vi "Dashboard Main.vi"() -> ()   [LabVIEW 2015]
uses:
  <vilib>/Utility/miscctls.llb/LVRowAndColumnTypeDef.ctl
  <vilib>/event_ctls.llb/eventvkey.ctl
  <vilib>/Rock Robotics/WPI/Dashboard/WPI_DashboardLogging Global.vi
  <vilib>/Rock Robotics/Network Tables/NT Read Boolean.vi
  <vilib>/Rock Robotics/Network Tables/NT Read Numeric Array.vi
  <vilib>/Utility/config.llb/Write Key (String).vi
  <vilib>/Utility/config.llb/Write Key (I32).vi
  <vilib>/Utility/config.llb/NI_LVConfig.lvlib
panel:
  in  "TCP":refnum<k5>
  in  "Rec Mode":enum32{"Stop", "Record", "Playback"}(radio)
  in  "Vision":u16(ring) items=["Camera Off", "USB Camera SW", "USB Camera HW", "IP Camera"]
  out "Camera IP":string
  out "Image Message":string="Timeout in Camera Communications"
  in  "Dashboard Tab":T1(tab)
  in  "Select Auto":string(combo)
  out "NT Connection":bool
  in  "Camera Settings":T2={"Frame Rate"=30, "Compression"=30, "Size"=1} {"Frame Rate" scale=1.0..30.0; "Size" items=["640x480", "320x240", "160x120"]}
  out "MotorChart R":cluster{"Numeric":dbl, "Numeric":dbl}(graph)
  out "MotorChart L":T3(graph)
  out "MotorSliders R":cluster{"MotorSlide1":dbl, "MotorSlide2":dbl} {"MotorSlide2" scale=-1.0..1.0 scale format="%#_2e"; "MotorSlide1" scale=-1.0..1.0 scale format="%#_2e"}
  out "MotorSliders L":T4 {"MotorSlide4 2" scale=0.0..14.0 scale format="%#_2e"; "MotorSlide2" scale=-1.0..1.0 scale format="%#_2e"; "MotorSlide1" scale=-1.0..1.0 scale format="%#_2e"}
  out "JS1 Z":dbl(slide) scale=-1.0..1.0 scale format="%#_2e"
  out "JS1 Graph":cluster{"X":dbl, "Y":dbl}[](graph)
  out "JS1 Buttons":T5
  out "JS2 Z":dbl(slide) scale=-1.0..1.0 scale format="%#_2e"
  out "JS2 Graph":cluster{"X":dbl, "Y":dbl}[](graph)
  out "JS2 Buttons":T5
  out "Mode":T6(ring)=enum."Auto Disabled"
  in  "DB Camera Config":bool
  out "fps":dbl format="%#.1g"
  out "Mbps":dbl format="%#.1g"
  out "Mbps LED":bool
  out "Accelerometre/temps":dbl(graph)
  in  "DB/String 9":string
  in  "DB/String 8":string
  in  "DB/String 7":string
  in  "DB/String 6":string
  in  "DB/String 5":string
  in  "DB/String 4":string
  in  "DB/String 3":string
  in  "DB/String 2":string
  in  "DB/String 1":string
  in  "DB/String 0":string
  in  "DB/Slider 0":dbl(slide) scale=0.0..5.0
  in  "DB/Slider 1":dbl(slide) scale=0.0..5.0
  in  "DB/Slider 2":dbl(slide) scale=0.0..5.0
  in  "DB/Slider 3":dbl(slide) scale=0.0..5.0
  out "DB/LED 3":bool
  out "DB/LED 2":bool
  out "DB/LED 1":bool
  out "DB/LED 0":bool
  in  "DB/Button 3":bool
  in  "DB/Button 2":bool
  in  "DB/Button 1":bool
  in  "DB/Button 0":bool caption="New Name"
  out "Voltage Right2":dbl
  out "Voltage Right1":dbl
  out "Voltage Left2":dbl
  out "Voltage Left1":dbl
  in  "vitesse gauche":dbl
  in  "temps de changement de direction":dbl=2.0
  in  "temps pleine vitesse":dbl=1.0
  in  "vitesse droit":dbl
  out "gauche rapide 2":bool
  out "gauche fort 2":bool
  out "droit rapide 2":bool
  out "droit fort  2":bool
  in  "Test Slider":dbl(slide) scale=0.0..100.0 scale format="%#_3g"
  in  "On/Off":bool caption="Solenoid"
  in  "Test Name":u16(ring) items=["Select the test to run..."]
  in  "Test Tree":string(tree)
  in  "Motor":cluster{"Value":dbl, "Enable":bool} {"Value" scale=-1.0..1.0 scale format="%#_3g"}
  out "Progress":T7 {"Test Progress" scale=0.0..100.0}
  in  "Rev/Fwd":cluster{"Forward":bool, "Reverse":bool}
  in  "Test Ring":u16(ring) items=["Monochrome", "Color"]
  out "Cmd Status":string
  in  "Execute Command":bool
  in  "Command Params":string[][](table)
  in  "Command Selection":i32(listbox)
  in  "CheckList":i32(listbox)
  out "Tree":string(tree)
  out "Camera Image":T8(plugin-control)
  out "Background":bool
  # "Left"
  # "Front"
  # "Right"
  # "Battery"
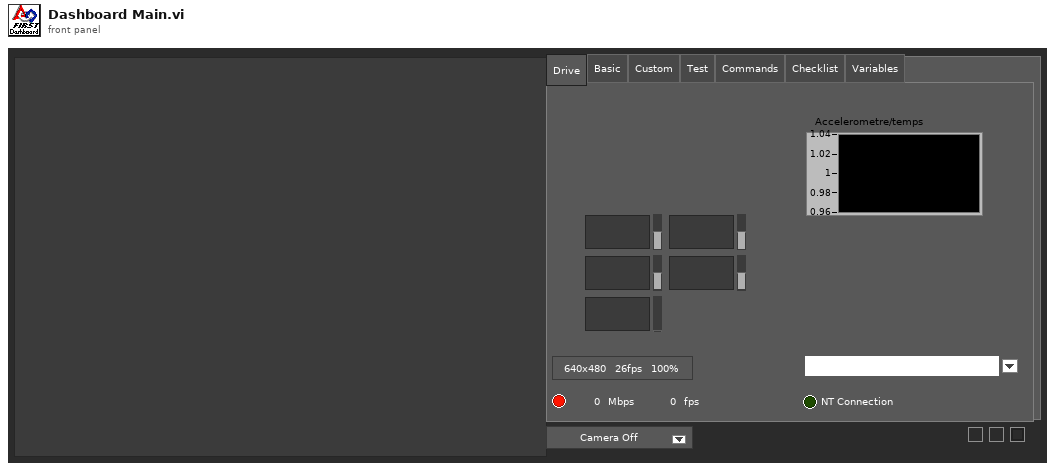
[diagram p1: front panel]
types:
  T1 = enum32{"Drive", "Basic", "Custom", "Test", "Commands", "Checklist", "Variables"}
  T2 = cluster{"Frame Rate":i32, "Compression":i32, "Size":u16}
  T3 = cluster{"Numeric":dbl, "Numeric":dbl, "Battery V":dbl}
  T4 = cluster{"MotorSlide1":dbl, "MotorSlide2":dbl, "MotorSlide4 2":dbl}
  T5 = cluster{bool, bool, bool, bool, bool, bool, bool, bool, bool, bool, bool, bool}
  T6 = enum8{"Tele-Op Disabled", "Tele-Op Enabled", "Auto Disabled", "Auto Enabled", "Test Disabled", "Test Enabled", "Disconnected", "No Code", "E-Stop"}
  T7 = cluster{"Test Progress":u8, "Test Progress Text":string}
  T8 = typedef "IMAQ Image.ctl" = refnum<image>
  T9 = cluster{"IDs":cluster{"RPC field ID":u16, "Unique ID":u16}, "String":string}
  T10 = enum32{"Drive", "Basic", "Custom", "Test", "Checklist", "Variables"}
  T11 = typedef "Image Type" = u32
  T12 = cluster{"Camera Image":refnum<vi>, "Dashboard Tab":refnum<vi>, "Background":refnum<vi>, "Vision":refnum<vi>, "Rec Mode":refnum<vi>, "Test Slider":refnum<vi>, "On/Off ":refnum<vi>, "Test Ring":refnum<vi>, "Rev/Fwd":refnum<vi>, "Test Name":refnum<vi>, "Motor":refnum<vi>, "Progress":refnum<vi>, "CheckList":refnum<vi>, "Tree":refnum<vi>, "Test Tree":refnum<vi>, "Command Params":refnum<vi>, "Command Selection":refnum<vi>, "Execute Command":refnum<vi>, "Cmd Status":refnum<vi>}
  T13 = cluster{"Error Strings":string, "Disable Counts":cluster{u16, u16}, "Rail Faults":cluster{u16, u16, u16}, "Robot IP":string, "DB Mode":u8, "Event Info":cluster{"Name":string, "Type":u8, "Number":u16, "Replay":u8}, "Camera Addr":string}
  T14 = cluster{"Storage":cluster{"Disk Free":u64, "RAM Block":u32, "RAM free":u32}, "CPU Utilization":cluster{"CPU % ISR":sgl, "CPU % Time Crit":sgl, "CPU % Timed Str":sgl, "CPU % High":sgl, "CPU % Above":sgl, "CPU % Normal":sgl, "CPU % Low":sgl}, "CAN":cluster{"% Bus Utilization":sgl, "Bus Off Cnt":u32, "TX_FIFO Full Cnt":u32, "Receive Error Cnt":u8, "Transmit Error Cnt":u8}, "HID":cluster{"HID Outputs":u32, "Rumble Low":u16, "Rumble High":u16}[]}
  T15 = cluster{"Status bits":cluster{"Test Mode":bool, "Autonomous":bool, "Enabled":bool, "Code Start":bool, "Brownout":bool, "Reserved 2":bool, "Reserved 3":bool, "E-Stop":bool}, "Code Trace":cluster{"Disabled":bool, "TeleOp":bool, "Auto":bool, "Test":bool}, "Controller Type":enum16{"unknown", "cRIO", "roboRio"}, "Code?":enum16{"unknown", "noCode", "code"}, "Battery V":dbl}
  T16 = cluster{"Control Bits":cluster{"TestMode":bool, "Autonomous":bool, "Enabled":bool, "FMS Present":bool, bool, bool, bool, "E-Stop":bool}, "Team Station ":u8, "Countdown":sgl, "Joystick Values":cluster{"Axes":dbl[], "Buttons":bool[], "POVs":i16[]}[]}
  T17 = cluster{"Axes":dbl[], "Buttons":bool[], "POVs":i16[]}[]
  T18 = cluster{"Axes":dbl[], "Buttons":bool[], "POVs":i16[]}
  T19 = cluster{"Buttons[0]":bool, "Buttons[1]":bool, "Buttons[2]":bool, "Buttons[3]":bool, "Buttons[4]":bool, "Buttons[5]":bool, "Buttons[6]":bool, "Buttons[7]":bool, "Buttons[8]":bool, "Buttons[9]":bool, "Buttons[10]":bool, "Buttons[11]":bool}
  T20 = typedef "NI_LVConfig.lvlib/Config Data RefNum.ctl" = refnum<k1>
  T21 = cluster{"Operation":enum16{"Update", "Clear"}, "Color Box":u32}[]
  T22 = typedef "eventvkey.ctl" = enum16{"ASCII", "Enter", "Return", "Shift", "Ctrl", "Alt", "Cmd", "Opt", "Caps", "NumLock", "Clear", "Break", "Up", "Down", "Left", "Right", "Insert", "Delete", "Home", "End", "PageUp", "PageDown", "Escape", "Help", "Pause", "ScrollLock", "F1", "F2", "F3", "F4", "F5", "F6", "F7", "F8", "F9", "F10", "F11", "F12", "F13", "F14", "F15", "F16", "F17", "F18", "F19", "F20", "F21", "F22", "F23", "F24", "Play", "VolumeUp", "VolumeDown", "Mute", "Two Byte Char"}
  T23 = cluster{"Image Size":bool, "Image Type":bool, "Pixel Value":bool, "ROI Information":bool, "Zoom Factor":bool}
  T24 = enum8{"Enabled", "Disabled", "Disabled and Grayed Out"}
  T25 = cluster{"Operation":enum16{"Update", "Clear"}, "Color Box":u32}
  T26 = typedef "LVRowAndColumnTypeDef.ctl" = cluster{"Row":i32, "Column":i32}
  T27 = cluster{"Shift":bool, "Ctrl":bool, "Alt":bool, "Cmd":bool, "Opt":bool}
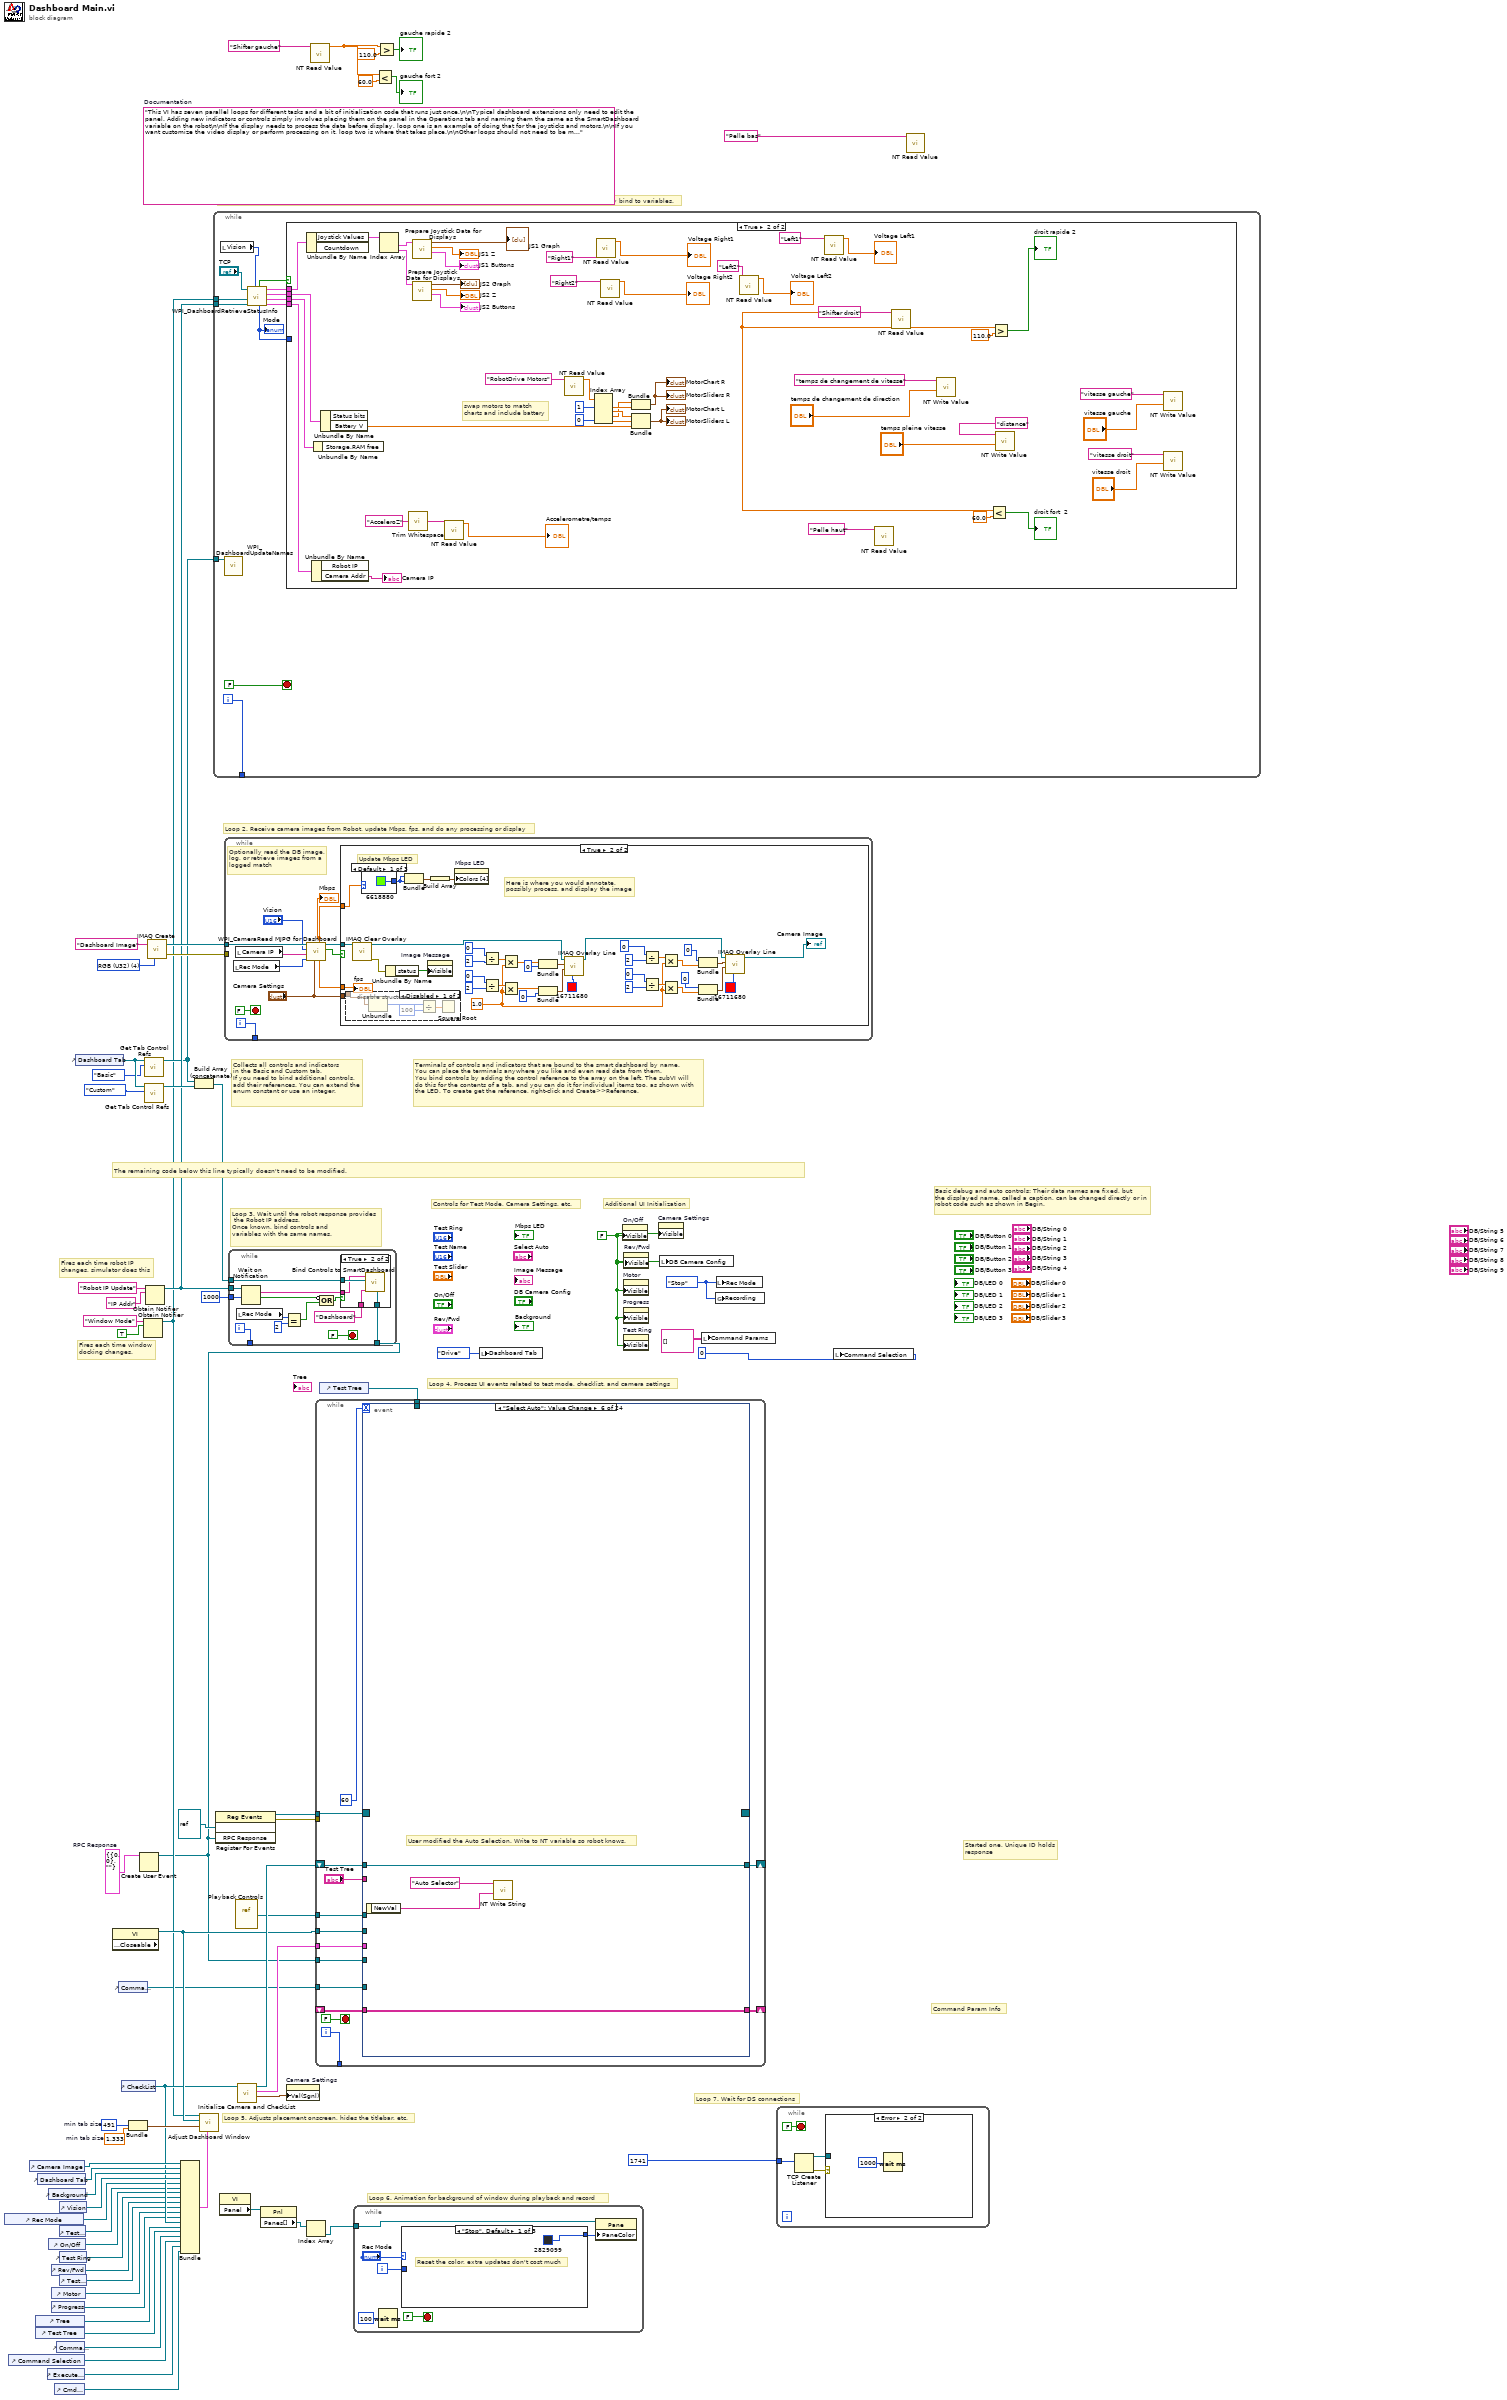
[diagram p0: block diagram]
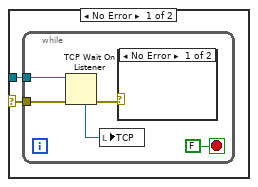
[diagram p2: hidden frame]
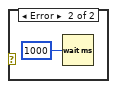
[diagram p3: hidden frame]
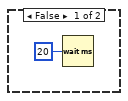
[diagram p4: hidden frame]
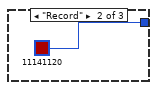
[diagram p5: hidden frame]
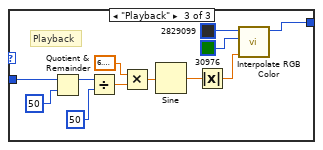
[diagram p6: hidden frame]
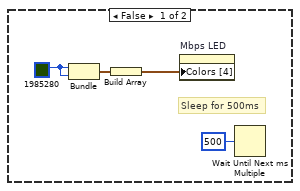
[diagram p8: hidden frame]
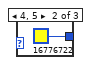
[diagram p10: hidden frame]
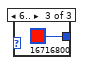
[diagram p11: hidden frame]
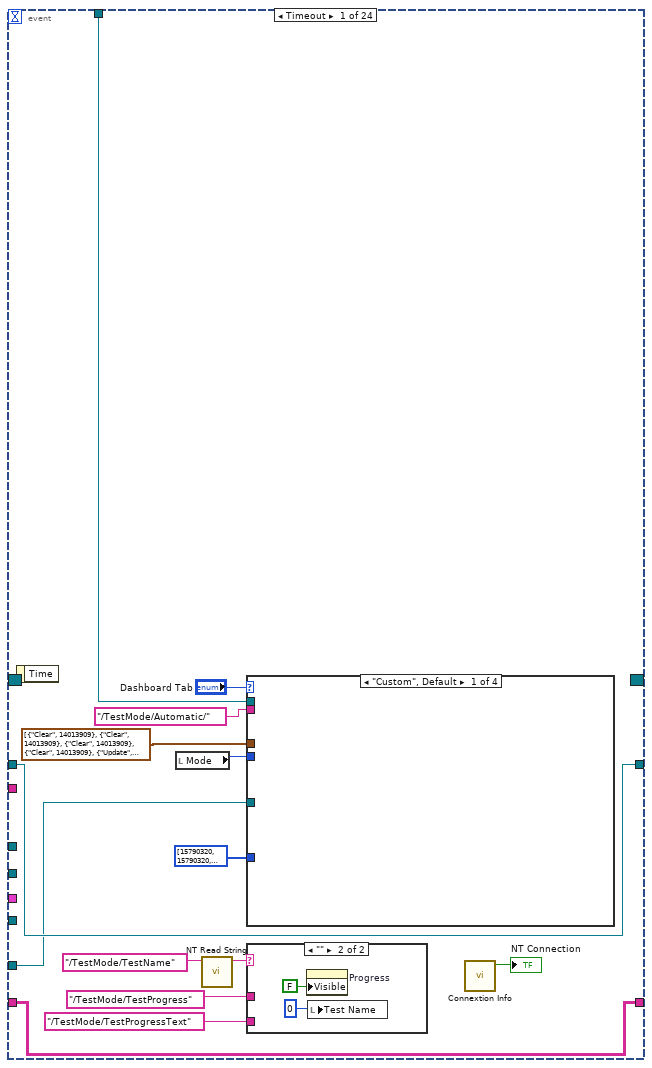
[diagram p12: hidden frame]
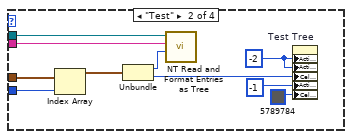
[diagram p13: hidden frame]
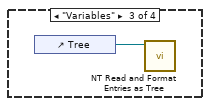
[diagram p14: hidden frame]
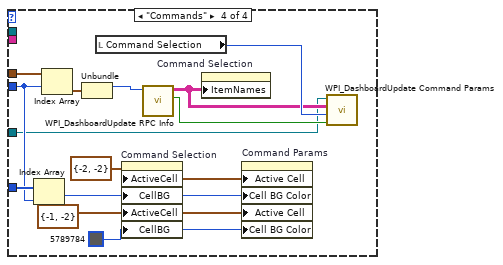
[diagram p15: hidden frame]
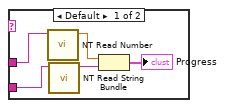
[diagram p16: hidden frame]
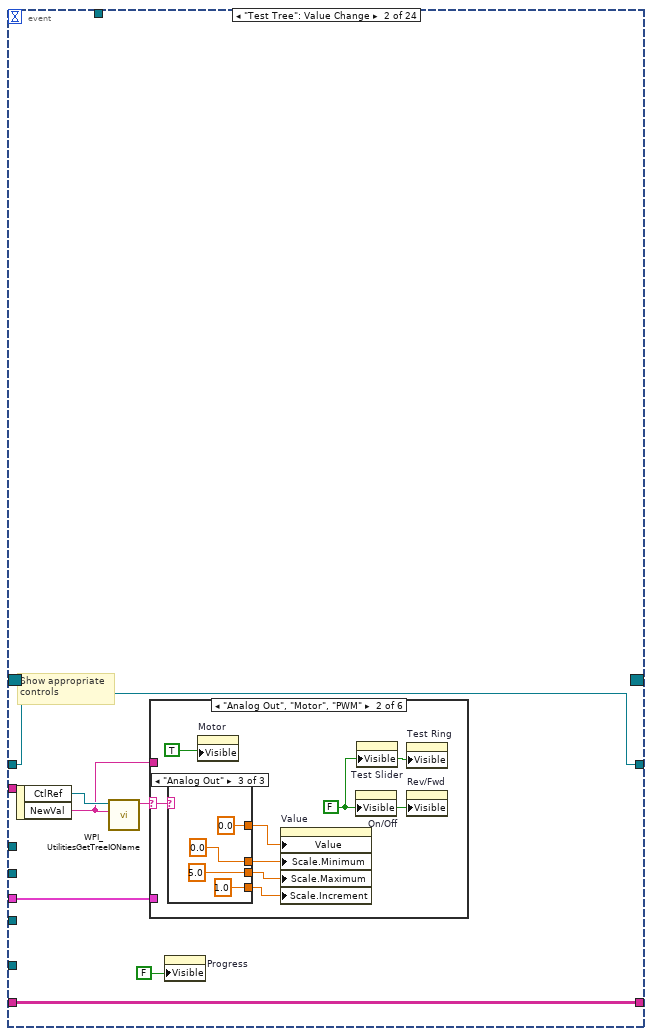
[diagram p17: hidden frame]
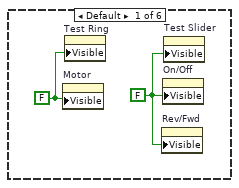
[diagram p18: hidden frame]
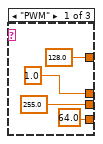
[diagram p19: hidden frame]
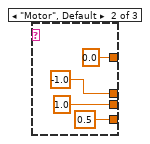
[diagram p20: hidden frame]
diagram:
  w14 = T9 {"IDs"={"RPC field ID"=0, "Unique ID"=0}, "String"=""}  # RPC Response
  w40 = 491  # min tab size
  w39 = 1.333  # min tab size
  w48 = enum32{"Stop", "Record", "Playback"}."Stop" ("Rec Mode")
  w22 = FALSE ("Visible")
  (unwired) "This VI has seven parallel loops for different tasks and a bit of initialization code that runs just once.\n\nTypical dashboard extensions only need to edit the panel. Adding new indicators or controls simply involves placing them on the panel in the Operations tab and naming them the same as the SmartDashboard variable on the robot\n\nIf the display needs to process the data before display, loop one is an example of doing that for the joysticks and motors.\n\nIf you want customize the video display or perform processing on it, loop two is where that takes place.\n\nOther loops should not need to be modified. They are pretty standard, and document the task they perform."  # Documentation
  w68 = T11 4 items=["Grayscale (U8)", "Grayscale (I16)", "Grayscale (SGL)", "Complex (CSG)", "RGB (U32)", "HSL (U32)", "RGB (U64)"] ("Image Type")
  # "Command Param Info"
  # "Started one, Unique ID holds\nresponse"
  # "Loop 7. Wait for DS connections"
  # "Basic debug and auto controls: Their data names are fixed, but\nthe displayed name, called a caption, can be changed directly or in\nrobot code such as shown in Begin."
  # "Controls for Test Mode, Camera Settings, etc."
  # "Additional UI Initialization"
  # "Loop 6. Animation for background of window during playback and record"
  # "Fires each time robot IP\nchanges, simulator does this"
  # "Fires each time window\ndocking changes."
  # "Collects all controls and indicators\nin the Basic and Custom tab.\nIf you need to bind additional controls,\nadd their references. You can extend the\nenum constant or use an integer."
  # "The remaining code below this line typically doesn't need to be modified."
  # "Loop 4. Process UI events related to test mode, checklist, and camera settings"
  # "Terminals of controls and indicators that are bound to the smart dashboard by name.\nYou can place the terminals anywhere you like and even read data from them.\nYou bind controls by adding the control reference to the array on the left. The subVI will\ndo this for the contents of a tab, and you can do it for individual items too, as shown with\nthe LED. To create get the reference, right-click and Create>>Reference."
  # "Loop 3. Wait until the robot response provides\n the Robot IP address.\nOnce known, bind controls and\nvariables with the same names."
  # "Loop 5. Adjusts placement onscreen, hides the titlebar, etc."
  # "Loop 1. Receive various data streams from Driver Station, update joystick, motors, and more complex displays that don't easily bind to variables."
  # "Loop 2. Receive camera images from Robot, update Mbps, fps, and do any processing or display"
  n1 = control-ref of="Rec Mode"() -> (w28:refnum<vi>)
  n2 = control-ref of="Command Selection"() -> (w13:refnum<vi>)
  n3 = control-ref of="Camera Image"() -> (w43:refnum<vi>)
  n4 = control-ref of="Tree"() -> (w32:refnum<vi>)
  n5 = control-ref of="Test Tree"() -> (w31:refnum<vi>)
  n6 = control-ref of="Dashboard Tab"() -> (w42:refnum<vi>)
  n7 = control-ref of="Execute Command"() -> (w15:refnum<vi>)
  n8 = control-ref of="Background"() -> (w37:refnum<vi>)
  n9 = control-ref of="On/Off"() -> (w26:refnum<vi>)
  n10 = control-ref of="Progress"() -> (w23:refnum<vi>)
  n11 = control-ref of="Rev/Fwd"() -> (w24:refnum<vi>)
  n12 = control-ref of="Motor"() -> (w29:refnum<vi>)
  n13 = control-ref of="Cmd Status"() -> (w9:refnum<vi>)
  n14 = control-ref of="Command Params"() -> (w16:refnum<vi>)
  n15 = control-ref of="Test Slider"() -> (w27:refnum<vi>)
  n16 = control-ref of="Vision"() -> (w41:refnum<vi>)
  n17 = control-ref of="Test Ring"() -> (w25:refnum<vi>)
  n18 = control-ref of="Test Name"() -> (w30:refnum<vi>)
  n19 = control-ref of="Dashboard Tab"() -> (w46:refnum<vi>)
  n20 = property class="VI" props=["Front Panel.Closeable"]() -> (reference out=w47:refnum<vi>)  [unwired: 2 in, 2 out]
  n21 = control-ref of="Command Params"() -> (w8:refnum<vi>)
  n22 = control-ref of="CheckList"() -> (w33:refnum<vi>)
  n23 = Bundle("min tab size"=w40, "min tab size"=w39) -> (w38:cluster{"min tab size":i32, "min tab size":dbl})  [unwired: 1 in]
  n24 = Create User Event(user event datatype=w14) -> (user event=w10:refnum<user-event>)  [unwired: 1 in, 1 out]
  n25 = Obtain Notifier(name (unnamed)="Window Mode", notification data type=TRUE) -> (notifier out=w19:refnum<notifier>)  [unwired: 2 in, 2 out]
  n26 = call <vilib>:"Get Tab Control Refs.vi"("Page Index"=T10."Basic" ("Dashboard Tab"), "TabControl in"=w46) -> ("ControlsOnPage"=w20:refnum<vi>[])  [unwired: 9 in]
  n27 = call <vilib>:"Get Tab Control Refs.vi"("Page Index"=T10."Custom" ("Dashboard Tab"), "TabControl in"=w46) -> ("ControlsOnPage"=w45:refnum<vi>[])  [unwired: 9 in]
  n28 = Obtain Notifier(name (unnamed)="Robot IP Update", notification data type="IP Addr" ("name (unnamed)")) -> (notifier out=w21:refnum<notifier>)  [unwired: 2 in, 2 out]
  n29 = call "IMAQ Create"("Image Name"="Dashboard Image", "Image Type"=w68) -> ("New Image"=w66:T8, "error out"=w65:errorcluster)  [unwired: 2 in, 1 out]
  n30 = Bundle("Camera Image"=w43, "Dashboard Tab"=w42, "Background"=w37, "Vision"=w41, "Rec Mode"=w28, "Test Slider"=w27, "On/Off"=w26, "Test Ring"=w25, "Rev/Fwd"=w24, "Test Name"=w30, "Motor"=w29, "Progress"=w23, "CheckList"=w33, "Tree"=w32, "Test Tree"=w31, "Command Params"=w16, "Command Selection"=w13, "Execute Command"=w15, "Cmd Status"=w9) -> (w34:T12)  [unwired: 1 in]
  n31 = Build Array (concatenate)(w20, w45) -> (w44:refnum<vi>[])
  n32 = call "Adjust Dashboard Window.vi"("Sizing Refnums"=w34, "Size Constraints"=w38, "VI"=w47, "WIn Mode"=w19) -> ()  [unwired: 8 in]
  n33 = while {
    tunnel: [w80] -> _
    tunnel: w21 -> [w74]
    tunnel: w20 -> [w73]
    tunnel: w19 -> [w69]
    i -> [w80]
    stop <- FALSE stop-if-true
    n34 = local read "Vision"() -> (w71:u16)
    n35 = call <vilib>:"WPI_DashboardUpdateNames.vi"("Controls on Tab"=w73) -> ()  [unwired: 11 in]
    n36 = call <vilib>:"WPI_DashboardRetrieveStatusInfo.vi"("Vision"=w71, "Binding Refnum"=w74, "Window Mode Notifier"=w69, "TCP Cnx"="TCP") -> ("Power and Errors"=w75:T13, "Robot Metrics"=w78:T14, "Status Info"=w79:T15, "Control Info"=w76:T16, "Robot Mode"=w72:T6, "Process?"=w77:bool)  [unwired: 2 in]
    "Mode" <- w72
    n37 = case shown="True" w77 {
      tunnel: w79 -> [_ w133]
      tunnel: w78 -> [_ w132]
      tunnel: w76 -> [_ w131]
      tunnel: w75 -> [_ w130]
      tunnel: w72 -> [_ _]
      frame False {
        n38 = Wait (ms)(milliseconds to wait=u32 20) -> ()  [unwired: 1 out]
      }
      frame True {
        # "swap motors to match\ncharts and include battery"
        n39 = Unbundle By Name(w131) -> ("Joystick Values"=w120:T17)  [unwired: 1 out]
        n40 = Unbundle By Name(w130) -> ("Camera Addr"=→"Camera IP":string)  [unwired: 1 out]
        n41 = Unbundle By Name(w132) -> ()  [unwired: 1 out]
        n42 = Unbundle By Name(w133) -> ("Battery V"=w121:dbl)  [unwired: 1 out]
        n43 = Index Array(array=w120) -> (element #1=w119:T18, element #2=w114:T18)  [unwired: 2 in]
        n44 = call <vilib>:"Trim Whitespace.vi"("string"="AcceleroZ") -> ("trimmed string"=w93:string)  [unwired: 1 in]
        n45 = call "Prepare Joystick Data for Displays.vi"("Joystick Values"=w114) -> ("Buttons"=→"JS2 Buttons":T19, "Z Axis"=→"JS2 Z":dbl, "Cartesian Data"=→"JS2 Graph":cluster{"X axis":dbl, "X axis":dbl}[])  [unwired: 8 in]
        n46 = call "Prepare Joystick Data for Displays.vi"("Joystick Values"=w119) -> ("Buttons"=→"JS1 Buttons":T19, "Z Axis"=→"JS1 Z":dbl, "Cartesian Data"=→"JS1 Graph":cluster{"X axis":dbl, "X axis":dbl}[])  [unwired: 8 in]
        n47 = call-poly <vilib>:"NT Read Value.vi"("Name"=w93) -> ("Numeric"=→"Accelerometre/temps":dbl)  [unwired: 9 in, 1 out]
        n48 = call-poly <vilib>:"NT Read Value.vi"("Name"="RobotDrive Motors") -> ("Numeric Array"=w109:dbl[])  [unwired: 9 in, 1 out]
        n49 = Index Array(array=w109, index #1=1, index #4=0) -> (element #1=w125:dbl, element #2=w126:dbl, element #3=w124:dbl, element #4=w129:dbl)  [unwired: 2 in]
        n50 = call-poly <vilib>:"NT Read Value.vi"("Name"="Right1") -> ("Numeric"=→"Voltage Right1":dbl)  [unwired: 9 in, 1 out]
        n51 = call-poly <vilib>:"NT Read Value.vi"("Name"="Right2") -> ("Numeric"=→"Voltage Right2":dbl)  [unwired: 9 in, 1 out]
        n52 = Bundle("Numeric"=w124, "Numeric"=w125) -> (→"MotorChart R" →"MotorSliders R":cluster{"Numeric":dbl, "Numeric":dbl})  [unwired: 1 in]
        n53 = Bundle("Numeric"=w126, "Numeric"=w129, "Battery V"=w121) -> (→"MotorChart L" →"MotorSliders L":T3)  [unwired: 1 in]
        n54 = call-poly <vilib>:"NT Read Value.vi"("Name"="Left2") -> ("Numeric"=→"Voltage Left2":dbl)  [unwired: 9 in, 1 out]
        n55 = call-poly <vilib>:"NT Read Value.vi"("Name"="Left1") -> ("Numeric"=→"Voltage Left1":dbl)  [unwired: 9 in, 1 out]
        n56 = call-poly <vilib>:"NT Read Value.vi"("Name"="Pelle haut") -> ()  [unwired: 9 in, 2 out]
        n57 = call-poly <vilib>:"NT Read Value.vi"("Name"="Shifter droit") -> ("Numeric"=w99:dbl)  [unwired: 9 in, 1 out]
        n58 = call-poly <vilib>:"NT Write Value.vi"("Numeric"="temps de changement de direction", "Name"="temps de changement de vitesse") -> ()  [unwired: 9 in, 1 out]
        n59 = Less?(x=w99, y=60.0) -> (x < y?=→"droit fort  2":bool)
        n60 = Greater?(x=w99, y=110.0) -> (0:→"droit rapide 2":bool)
        n61 = call-poly <vilib>:"NT Write Value.vi"("Numeric"="temps pleine vitesse", "Name"="distance") -> ()  [unwired: 9 in, 1 out]
        n62 = call-poly <vilib>:"NT Write Value.vi"("Numeric"="vitesse gauche", "Name"="vitesse gauche") -> ()  [unwired: 9 in, 1 out]
        n63 = call-poly <vilib>:"NT Write Value.vi"("Numeric"="vitesse droit", "Name"="vitesse droit") -> ()  [unwired: 9 in, 1 out]
      }
    }
  }
  n64 = register-events(refnum<vi> refnum, w10) -> (reference out=w52:refnum<event-registration>, error out=w51:errorcluster)  [unwired: 2 in]
  n65 = property class="VI"() -> ("Panel"=w55:refnum<vi>)  [unwired: 2 in, 2 out]
  n66 = while {
    tunnel: w66 -> [w142]
    tunnel: w65 -> [_]
    tunnel: [w143] -> _
    i -> [w143]
    stop <- FALSE stop-if-true
    # "Optionally read the DB image,\nlog, or retrieve images from a\nlogged match"
    n67 = local read "Rec Mode"() -> (w138:enum32{"Stop", "Record", "Playback"})
    n68 = local read "Camera IP"() -> (w136:string)
    n69 = call <vilib>:"WPI_CameraRead MJPG for Dashboard.vi"("Camera Settings"="Camera Settings", "Rec Mode"=w138, "Camera IP"=w136, "Camera Mode"="Vision", "Refnum in"=w142) -> ("Active"=w140:bool, "Refnum out"=w141:T8, "FPS"=w139:dbl, "Bandwidth (Mbps)"=w135:dbl)  [unwired: 3 in]
    "Mbps" <- w135
    n70 = case shown="True" w140 {
      tunnel: w141 -> [_ w182]
      tunnel: w135 -> [_ w181]
      tunnel: w139 -> [_ w180]
      tunnel: "Camera Settings" -> [_ w178]
      frame False {
        w145 = u32 1985280 ("Color Box")
        # "Sleep for 500ms"
        n71 = Bundle("Color Box"=w145, "Color Box"=w145) -> (w147:cluster{"Color Box":u32, "Color Box":u32})  [unwired: 1 out]
        n72 = Build Array(w147) -> (w146:cluster{"Color Box":u32, "Color Box":u32}[])
        n73 = property on="Mbps LED" class="Bool (strict)"("Colors [4]"=w146) -> ()  [unwired: 2 in, 2 out]
        n74 = Wait Until Next ms Multiple(millisecond multiple=u32 500) -> ()  [unwired: 1 out]
      }
      frame True {
        w149 = 1.0
        # "Here is where you would annotate,\npossibly process, and display the image"
        # "Update Mbps LED"
        n75 = disable-structure shown="Disabled" {
          disable-tunnel: w178 -> [w191 _]
          frame Disabled {
            n76 = Unbundle(w191) -> ("Compression"=w190:i32)  [unwired: 2 out]
            n77 = Divide(x=w190, y=100) -> (x/y=w188:dbl)
            n78 = Square Root(x=w188) -> ()  [unwired: 1 out]
          }
          frame Enabled {
          }
        }
        n79 = call "IMAQ Clear Overlay"("Image"=w182) -> ("error out"=w186:errorcluster, "Image Out"=w179:T8)  [unwired: 2 in, 7 out]
        n80 = case shown="Default" w181 {
          tunnel: [u32 6618880 ("Color Box") u32 16776722 ("Color Box") u32 16716800 ("Color Box")] -> w183
          frame Default {
          }
          frame 4, 5 {
          }
          frame 6.. {
          }
        }
        n81 = Unbundle By Name(w186) -> ("status"=w187:bool)
        n82 = Bundle("Color Box"=w183, "Color Box"=w183) -> (w185:cluster{"Color Box":u32, "Color Box":u32})  [unwired: 1 out]
        n83 = property on="Image Message" class="Str"("Visible"=w187) -> ()  [unwired: 2 in, 2 out]
        n84 = Build Array(w185) -> (w184:cluster{"Color Box":u32, "Color Box":u32}[])
        n85 = property on="Mbps LED" class="Bool (strict)"("Colors [4]"=w184) -> ()  [unwired: 2 in, 2 out]
        n86 = Divide(x=0, y=2) -> (x/y=w174:dbl)
        n87 = Divide(x=0, y=2) -> (x/y=w169:dbl)
        n88 = Multiply(x=w174, y=w149) -> (x*y=w173:dbl)
        n89 = Multiply(x=w169, y=w149) -> (x*y=w168:dbl)
        n90 = Bundle(w173, 0) -> (w177:cluster{dbl, i32})  [unwired: 1 in]
        n91 = Bundle(w168, 0) -> (w166:cluster{dbl, i32})  [unwired: 1 in]
        n92 = call "IMAQ Overlay Line"("Color"=u32 16711680, "End Point"=w166, "Start Point"=w177, "Image"=w179) -> ("Image Out"=w157:T8)  [unwired: 6 in, 1 out]
        n93 = Divide(x=0, y=2) -> (x/y=w162:dbl)
        n94 = Divide(x=0, y=2) -> (x/y=w159:dbl)
        n95 = Multiply(x=w162, y=w149) -> (x*y=w155:dbl)
        n96 = Multiply(x=w159, y=w149) -> (x*y=w153:dbl)
        n97 = Bundle(0, w155) -> (w165:cluster{i32, dbl})  [unwired: 1 in]
        n98 = Bundle(0, w153) -> (w158:cluster{i32, dbl})  [unwired: 1 in]
        n99 = call "IMAQ Overlay Line"("Color"=u32 16711680, "End Point"=w158, "Start Point"=w165, "Image"=w157) -> ("Image Out"=→"Camera Image":T8)  [unwired: 6 in, 1 out]
        "fps" <- w180
      }
    }
  }
  n100 = while {
    tunnel: w44 -> [w207]
    tunnel: w21 -> [w205]
    tunnel: [w203] -> _
    tunnel: u32 1000 ("milliseconds to wait") -> [w202]
    tunnel: w10 -> [w195]
    i -> [w203]
    stop <- FALSE stop-if-true
    n101 = local read "Rec Mode"() -> (w198:enum32{"Stop", "Record", "Playback"})
    n102 = Wait on Notification(notifier=w205, timeout in ms (-1)=w202) -> (notification=w204:string, timed out?=w200:bool)  [unwired: 2 in, 2 out]
    n103 = Equal?(x=w198, y=u16 2 ("Rec Mode")) -> (x = y?=w199:bool)
    n104 = Compound Arithmetic op=OR(invert w200, w199) -> (w201:bool)
    n105 = case shown="True" w201 {
      tunnel: w207 -> [_ w211]
      tunnel: w204 -> [_ w210]
      tunnel: "Dashboard" -> [_ w209]
      tunnel: w195 -> [_ w208]
      frame False {
      }
      frame True {
        n106 = call <vilib>:"Bind Controls to SmartDashboard.vi"("RPC ref"=w208, "Client Name"=w209, "Bound Control Refs"=w211, "Server IP Address"=w210) -> ()  [unwired: 8 in]
      }
    }
  }
  n107 = vi-ref "Playback Controls.vi"() -> (w53:refnum<vi>)
  n108 = call "Initialize Camera and CheckList.vi"("ListBox in"=w33) -> ("Cluster"=w59:cluster{"value":i32, "value":i32, "index":i32}, "Array"=w60:cluster{string[]}[], "File Refnum"=w58:T20)  [unwired: 8 in]
  n109 = property class="Pnl"(reference=w55) -> ("Panes[]"=w56:refnum<vi>[])  [unwired: 1 in, 2 out]
  n110 = property on="Camera Settings" class="Clust (strict)"("Val(Sgnl)"=w59) -> ()  [unwired: 2 in, 2 out]
  n111 = Index Array(array=w56) -> (element=w54:refnum<vi>)  [unwired: 1 in]
  n112 = call-poly <vilib>:"NT Read Value.vi"("Name"="Shifter gauche") -> ("Numeric"=w4:dbl)  [unwired: 9 in, 1 out]
  n113 = control-ref of="Test Tree"() -> (w57:refnum<vi>)
  n114 = while {
    tunnel: w60 -> [w223]
    shift-right: [w222] -> _
    shift-left: w58 -> [w221]
    tunnel: [w220] -> _
    tunnel: w57 -> [w219]
    tunnel: w53 -> [w218]
    tunnel: w52 -> [w217]
    tunnel: w51 -> [_]
    tunnel: w47 -> [w216]
    tunnel: w10 -> [w215]
    tunnel: w8 -> [w214]
    shift-right: [w213] -> _
    shift-left: _ -> [w212]
    i -> [w220]
    stop <- FALSE stop-if-true
    n115 = event shown="[5] \"Select Auto\": Value Change" {
      selector: w217 -> [_ _ _ _ _ _ _ _ _ _ _ _ _ _ _ _ _ _ _ _ _ _ _ _]
      dyn-events: [_ _ _ _ _ _ _ _ _ _ _ _ _ _ _ _ _ _ w532 _ _ _ _ _] -> _
      timeout: u32 60 ("milliseconds to wait") -> [_ _ _ _ _ _ _ _ _ _ _ _ _ _ _ _ _ _ _ _ _ _ _ _]
      tunnel: w219 -> [w236 _ _ _ _ _ _ _ _ _ _ _ _ _ _ _ _ _ _ _ _ _ _ _]
      tunnel: "Test Tree" -> [_ _ _ _ _ _ _ _ _ _ _ _ _ w495 w504 w507 w512 w521 _ _ _ _ _ _]
      tunnel: w223 -> [_ w274 _ _ _ _ _ _ _ _ _ w457 w488 _ _ _ _ _ _ _ _ _ _ _]
      tunnel: [w233 w273 w377 w383 w393 w397 w403 w415 w423 w429 w442 w456 w481 w494 w502 w506 w511 w520 w534 w550 w552 w560 w571 w576] -> w222
      tunnel: w221 -> [w233 w273 w377 w383 w393 w397 w403 w415 w423 w429 w442 w455 w481 w494 w502 w506 w511 w520 w534 w550 w552 w560 w571 w576]
      tunnel: w218 -> [_ _ _ _ _ _ _ _ _ _ _ _ _ _ _ _ _ _ w535 _ w555 _ _ _]
      tunnel: w216 -> [_ _ _ _ _ _ _ _ _ _ _ _ _ _ _ _ _ _ w530 _ _ _ _ _]
      tunnel: w215 -> [_ _ _ _ _ _ _ _ _ _ _ _ _ _ _ _ _ _ w526 _ _ _ _ _]
      tunnel: w214 -> [w228 _ _ _ _ _ w401 _ _ _ _ _ _ _ _ _ _ _ _ _ _ _ _ _]
      tunnel: [w227 w272 w376 w382 w392 w398 w399 w409 w420 w428 w441 w454 w480 w493 w501 w505 w510 w519 w525 w548 w551 w556 w564 w577] -> w213
      tunnel: w212 -> [w227 w272 w376 w382 w392 w398 w399 _ _ w428 w441 w454 w480 w493 w501 w505 w510 w519 w525 w548 w551 w556 w564 w577]
      event Timeout {
        n116 = event-data() -> ()  [unwired: 1 in, 1 out]
        n117 = local read "Mode"() -> (w230:T6)
        n118 = call <vilib>:"NT Read String.vi"("Name"="/TestMode/TestName") -> ("String"=w239:string)  [unwired: 9 in, 1 out]
        n119 = case shown="\"Custom\", Default" "Dashboard Tab" {
          tunnel: w236 -> [_ w250 _ _]
          tunnel: "/TestMode/Automatic/" ("Name Pattern") -> [_ w249 _ _]
          tunnel: T21 [{"Operation"=enum."Clear", "Color Box"=14013909}, {"Operation"=enum."Clear", "Color Box"=14013909}, {"Operation"=enum."Clear", "Color Box"=14013909}, {"Operation"=enum."Clear", "Color Box"=14013909}, {"Operation"=enum."Update", "Color Box"=14013909}, {"Operation"=enum."Update", "Color Box"=16777215}, {"Operation"=enum."Clear", "Color Box"=14013909}, {"Operation"=enum."Clear", "Color Box"=14013909}, {"Operation"=enum."Clear", "Color Box"=14013909}] -> [_ w242 _ w259]
          tunnel: w230 -> [_ w241 _ w258]
          tunnel: u32[] [15790320, 15790320, 15790320, 15790320, 16777215, 16777215, 15790320, 15790320, 15790320] -> [_ _ _ w264]
          tunnel: w228 -> [_ _ _ w252]
          frame "Custom", Default {
          }
          frame "Test" {
            w248 = -2 ("Active Item:Row Number")
            n120 = Index Array(array=w242, index=w241) -> (element=w243:T25)
            n121 = Unbundle(w243) -> ("Operation"=w244:enum16{"Update", "Clear"}, "Color Box"=w245:u32)
            n122 = call <vilib>:"NT Read and Format Entries as Tree.vi"("Operation"=w244, "Name Pattern"=w249, "Tree Refnum"=w250) -> ()  [unwired: 7 in, 2 out]
            n123 = property on="Test Tree" class="Tree (strict)"("Active Item Row Number"=w248, "ActiveColNum"=w248, "CellBG"=w245, "Active Item Row Number"=-1 ("Active Item:Row Number"), "CellBG"=u32 5789784 ("Color Box")) -> ()  [unwired: 2 in, 2 out]
          }
          frame "Variables" {
            n124 = control-ref of="Tree"() -> (w251:refnum<vi>)
            n125 = call <vilib>:"NT Read and Format Entries as Tree.vi"("Tree Refnum"=w251) -> ()  [unwired: 9 in, 2 out]
          }
          frame "Commands" {
            w260 = u32 5789784 ("Color Box")
            w261 = T26 {"Row"=-1, "Column"=-2} ("Active Cell:Active Cell")
            w263 = T26 {"Row"=-2, "Column"=-2} ("Active Cell:Active Cell")
            n126 = Index Array(array=w264, index=w258) -> (element=w262:u32)
            n127 = Index Array(array=w259, index=w258) -> (element=w257:T25)
            n128 = Unbundle(w257) -> ("Operation"=w256:enum16{"Update", "Clear"})  [unwired: 1 out]
            n129 = local read "Command Selection"() -> (w255:i32)
            n130 = property on="Command Selection" class="MCListbox (strict)"("ActiveCell"=w263, "CellBG"=w262, "ActiveCell"=w261, "CellBG"=w260) -> ()  [unwired: 2 in, 2 out]
            n131 = call <vilib>:"WPI_DashboardUpdate RPC Info.vi"("Operation"=w256) -> ("update"=w254:bool, "commands"=w253:string[][])  [unwired: 9 in]
            n132 = property on="Command Selection" class="MCListbox (strict)"("ItemNames"=w253) -> ()  [unwired: 2 in, 2 out]
            n133 = property on="Command Params" class="Tbl (strict)"("Active Cell"=w263, "Cell BG Color"=w262, "Active Cell"=w261, "Cell BG Color"=w260) -> ()  [unwired: 2 in, 2 out]
            n134 = call <vilib>:"WPI_DashboardUpdate Command Params.vi"("Update"=w254, "NewVal"=w255, "Commands"=w253, "Param Tbl"=w252) -> ()  [unwired: 7 in, 1 out]
          }
        }
        n135 = case shown="\"\"" w239 {
          tunnel: "/TestMode/TestProgress" ("Name") -> [w266 _]
          tunnel: "/TestMode/TestProgressText" ("Name") -> [w265 _]
          frame Default {
            n136 = call <vilib>:"NT Read Number.vi"("Name"=w266) -> ("Numeric"=w267:dbl)  [unwired: 9 in, 1 out]
            n137 = call <vilib>:"NT Read String.vi"("Name"=w265) -> ("String"=w268:string)  [unwired: 9 in, 1 out]
            n138 = Bundle("Numeric"=w267, "String"=w268) -> (→"Progress":cluster{"Numeric":dbl, "String":string})  [unwired: 1 in]
          }
          frame "" {
            n139 = property on="Progress" class="Clust (strict)"("Visible"=FALSE) -> ()  [unwired: 2 in, 2 out]
            n140 = local write "Test Name"(u16 0) -> ()
          }
        }
        n141 = call <vilib>:"Connextion Info.vi"() -> ("Connected"=→"NT Connection":bool)  [unwired: 10 in, 1 out]
      }
      event "Test Tree": Value Change {
        # "Show appropriate\ncontrols"
        n142 = event-data() -> ("CtlRef"=w277:refnum<vi>, "NewVal"=w275:string)  [unwired: 1 in]
        n143 = call <vilib>:"WPI_UtilitiesGetTreeIOName.vi"("NewVal"=w275, "TreeControl in"=w277) -> ("I/O Name"=w278:string)  [unwired: 9 in]
        n144 = case shown="\"Analog Out\", \"Motor\", \"PWM\"" w278 {
          selector: w278 -> [_ w285 _ w307 w316 _]
          tunnel: w275 -> [_ _ w304 w306 _ w323]
          tunnel: w274 -> [_ _ _ _ _ w322]
          frame Default {
            w280 = FALSE ("Visible")
            w279 = FALSE ("Visible")
            n145 = property on="Motor" class="Clust (strict)"("Visible"=w279) -> ()  [unwired: 2 in, 2 out]
            n146 = property on="Test Ring" class="Ring (strict)"("Visible"=w279) -> ()  [unwired: 2 in, 2 out]
            n147 = property on="Rev/Fwd" class="Clust (strict)"("Visible"=w280) -> ()  [unwired: 2 in, 2 out]
            n148 = property on="On/Off" class="Bool (strict)"("Visible"=w280) -> ()  [unwired: 2 in, 2 out]
            n149 = property on="Test Slider" class="Slide (strict)"("Visible"=w280) -> ()  [unwired: 2 in, 2 out]
          }
          frame "Analog Out", "Motor", "PWM" {
            w286 = FALSE ("Visible")
            n150 = case shown="\"Analog Out\"" w285 {
              tunnel: [1.0 ("Value") -1.0 ("Value") 0.0 ("Value")] -> w284
              tunnel: [255.0 ("Value") 1.0 ("Value") 5.0 ("Value")] -> w283
              tunnel: [128.0 ("Value") 0.0 ("Value") 0.0 ("Value")] -> w282
              tunnel: [64.0 ("Value") 0.5 ("Value") 1.0 ("Value")] -> w281
              frame "PWM" {
              }
              frame "Motor", Default {
              }
              frame "Analog Out" {
              }
            }
            n151 = property on="Motor" class="Clust (strict)"("Visible"=TRUE) -> ()  [unwired: 2 in, 2 out]
            n152 = property on="Value" class="Slide (strict)"("Value"=w282, "Scale.Minimum"=w284, "Scale.Maximum"=w283, "Scale.Increment"=w281) -> ()  [unwired: 2 in, 2 out]
            n153 = property on="On/Off" class="Bool (strict)"("Visible"=w286) -> ()  [unwired: 2 in, 2 out]
            n154 = property on="Test Slider" class="Slide (strict)"("Visible"=w286) -> ()  [unwired: 2 in, 2 out]
            n155 = property on="Test Ring" class="Ring (strict)"("Visible"=w286) -> ()  [unwired: 2 in, 2 out]
            n156 = property on="Rev/Fwd" class="Clust (strict)"("Visible"=w286) -> ()  [unwired: 2 in, 2 out]
          }
          frame "Servo" {
            w302 = FALSE ("Visible")
            n157 = call <vilib>:"NT Read Number.vi"("Name"=w304) -> ("Numeric"=w303:dbl)  [unwired: 9 in, 1 out]
            n158 = property on="Test Slider" class="Slide (strict)"("Visible"=TRUE, "Scale.Maximum"=170.0 ("Scale.Range:Maximum")) -> ()  [unwired: 2 in, 2 out]
            n159 = local write "Test Slider"(w303) -> ()
            n160 = property on="Motor" class="Clust (strict)"("Visible"=w302) -> ()  [unwired: 2 in, 2 out]
            n161 = property on="Rev/Fwd" class="Clust (strict)"("Visible"=w302) -> ()  [unwired: 2 in, 2 out]
            n162 = property on="On/Off" class="Bool (strict)"("Visible"=w302) -> ()  [unwired: 2 in, 2 out]
            n163 = property on="Test Ring" class="Ring (strict)"("Visible"=w302) -> ()  [unwired: 2 in, 2 out]
          }
          frame "Relay", "Solenoid" {
            w305 = FALSE ("Visible")
            n164 = property on="Motor" class="Clust (strict)"("Visible"=w305) -> ()  [unwired: 2 in, 2 out]
            n165 = property on="Test Slider" class="Slide (strict)"("Visible"=w305) -> ()  [unwired: 2 in, 2 out]
            n166 = Search and Replace String(input string=w306, search string="/Value  **", replace string="/Direction") -> (result string=w312:string)  [unwired: 5 in, 3 out]
            n167 = property on="Test Ring" class="Ring (strict)"("Visible"=w305) -> ()  [unwired: 2 in, 2 out]
            n168 = call <vilib>:"NT Read String.vi"("Name"=w312) -> ("String"=w310:string)  [unwired: 9 in, 1 out]
            n169 = Equal?(x="Both directions", y=w310) -> (x = y?=w308:bool)
            n170 = Not(x=w308) -> (.not. x?=w309:bool)
            n171 = property on="Rev/Fwd" class="Clust (strict)"("Visible"=w308) -> ()  [unwired: 2 in, 2 out]
            n172 = property on="On/Off" class="Bool (strict)"("Visible"=w309, "Caption.Text"=w307) -> ()  [unwired: 2 in, 2 out]
          }
          frame "Compressor", "Digital Out" {
            w315 = FALSE ("Visible")
            # "Get direction and finish"
            n173 = property on="Motor" class="Clust (strict)"("Visible"=w315) -> ()  [unwired: 2 in, 2 out]
            n174 = property on="Test Slider" class="Slide (strict)"("Visible"=w315) -> ()  [unwired: 2 in, 2 out]
            n175 = property on="Test Ring" class="Ring (strict)"("Visible"=w315) -> ()  [unwired: 2 in, 2 out]
            n176 = property on="On/Off" class="Bool (strict)"("Visible"=TRUE, "Caption.Text"=w316) -> ()  [unwired: 2 in, 2 out]
            n177 = property on="Rev/Fwd" class="Clust (strict)"("Visible"=FALSE) -> ()  [unwired: 2 in, 2 out]
          }
          frame "Camera" {
            n178 = call <vilib>:"Get Last Path Segment.vi"("String in"=w323) -> ("String out"=w324:string)  [unwired: 10 in]
            n179 = property on="On/Off" class="Bool (strict)"("Visible"=FALSE) -> ()  [unwired: 2 in, 2 out]
            n180 = property on="Motor" class="Clust (strict)"("Visible"=FALSE) -> ()  [unwired: 2 in, 2 out]
            n181 = property on="Rev/Fwd" class="Clust (strict)"("Visible"=FALSE) -> ()  [unwired: 2 in, 2 out]
            n182 = case shown="\"White Balance  **\"" w324 {
              tunnel: w323 -> [w330 w339 w348 w357 w366 _ w372]
              tunnel: w322 -> [w328 w336 w345 w354 w363 _ _]
              frame "Size  **" {
                n183 = Index Array(array=w328) -> (element=w327:cluster{string[]})  [unwired: 1 in]
                n184 = call <vilib>:"NT Read String.vi"("Name"=w330) -> ("String"=w329:string)  [unwired: 9 in, 1 out]
                n185 = Unbundle(w327) -> (w325:string[])
                n186 = Match First String(2:w325, 3:w329) -> (0:w326:i32)  [unwired: 1 out]
                n187 = property on="Test Ring" class="Ring (strict)"("Value"=w326, "Strings []"=w325) -> ()  [unwired: 2 in, 2 out]
                n188 = property on="Test Ring" class="Ring (strict)"("Visible"=TRUE) -> ()  [unwired: 2 in, 2 out]
                n189 = property on="Test Slider" class="Slide (strict)"("Visible"=FALSE) -> ()  [unwired: 2 in, 2 out]
              }
              frame "White Balance  **" {
                n190 = Index Array(array=w336, index=1) -> (element=w337:cluster{string[]})
                n191 = call <vilib>:"NT Read String.vi"("Name"=w339) -> ("String"=w338:string)  [unwired: 9 in, 1 out]
                n192 = Unbundle(w337) -> (w334:string[])
                n193 = Match First String(2:w334, 3:w338) -> (0:w333:i32)  [unwired: 1 out]
                n194 = property on="Test Ring" class="Ring (strict)"("Value"=w333, "Strings []"=w334) -> ()  [unwired: 2 in, 2 out]
                n195 = property on="Test Ring" class="Ring (strict)"("Visible"=TRUE) -> ()  [unwired: 2 in, 2 out]
                n196 = property on="Test Slider" class="Slide (strict)"("Visible"=FALSE) -> ()  [unwired: 2 in, 2 out]
              }
              frame "Exposure  **" {
                n197 = Index Array(array=w345, index=2) -> (element=w346:cluster{string[]})
                n198 = call <vilib>:"NT Read String.vi"("Name"=w348) -> ("String"=w347:string)  [unwired: 9 in, 1 out]
                n199 = Unbundle(w346) -> (w342:string[])
                n200 = Match First String(2:w342, 3:w347) -> (0:w343:i32)  [unwired: 1 out]
                n201 = property on="Test Ring" class="Ring (strict)"("Value"=w343, "Strings []"=w342) -> ()  [unwired: 2 in, 2 out]
                n202 = property on="Test Ring" class="Ring (strict)"("Visible"=TRUE) -> ()  [unwired: 2 in, 2 out]
                n203 = property on="Test Slider" class="Slide (strict)"("Visible"=FALSE) -> ()  [unwired: 2 in, 2 out]
              }
              frame "Exposure Priority  **" {
                n204 = Index Array(array=w354, index=3) -> (element=w355:cluster{string[]})
                n205 = call <vilib>:"NT Read String.vi"("Name"=w357) -> ("String"=w356:string)  [unwired: 9 in, 1 out]
                n206 = Unbundle(w355) -> (w351:string[])
                n207 = Match First String(2:w351, 3:w356) -> (0:w352:i32)  [unwired: 1 out]
                n208 = property on="Test Ring" class="Ring (strict)"("Value"=w352, "Strings []"=w351) -> ()  [unwired: 2 in, 2 out]
                n209 = property on="Test Ring" class="Ring (strict)"("Visible"=TRUE) -> ()  [unwired: 2 in, 2 out]
                n210 = property on="Test Slider" class="Slide (strict)"("Visible"=FALSE) -> ()  [unwired: 2 in, 2 out]
              }
              frame "Color Enable  **" {
                n211 = Index Array(array=w363, index=4) -> (element=w364:cluster{string[]})
                n212 = call <vilib>:"NT Read String.vi"("Name"=w366) -> ("String"=w365:string)  [unwired: 9 in, 1 out]
                n213 = Unbundle(w364) -> (w360:string[])
                n214 = Match First String(2:w360, 3:w365) -> (0:w361:i32)  [unwired: 1 out]
                n215 = property on="Test Ring" class="Ring (strict)"("Value"=w361, "Strings []"=w360) -> ()  [unwired: 2 in, 2 out]
                n216 = property on="Test Ring" class="Ring (strict)"("Visible"=TRUE) -> ()  [unwired: 2 in, 2 out]
                n217 = property on="Test Slider" class="Slide (strict)"("Visible"=FALSE) -> ()  [unwired: 2 in, 2 out]
              }
              frame Default {
                n218 = property on="Test Ring" class="Ring (strict)"("Visible"=FALSE) -> ()  [unwired: 2 in, 2 out]
                n219 = property on="Test Slider" class="Slide (strict)"("Visible"=FALSE) -> ()  [unwired: 2 in, 2 out]
              }
              frame "Brightness  **", "Color Level  **", "Compression  **", "FPS  **", "Sharpness  **" {
                n220 = call <vilib>:"NT Read Number.vi"("Name"=w372) -> ("Numeric"=w371:dbl)  [unwired: 9 in, 1 out]
                n221 = local write "Test Slider"(w371) -> ()
                n222 = property on="Test Slider" class="Slide (strict)"("Visible"=TRUE, "Scale.Maximum"=100.0 ("Scale.Range:Maximum")) -> ()  [unwired: 2 in, 2 out]
                n223 = property on="Test Ring" class="Ring (strict)"("Visible"=FALSE) -> ()  [unwired: 2 in, 2 out]
              }
            }
          }
        }
        n224 = property on="Progress" class="Clust (strict)"("Visible"=FALSE) -> ()  [unwired: 2 in, 2 out]
      }
      event "Test Name": Mouse Enter {
        # "Populate the ring with the list of tests"
        n225 = event-data() -> ()  [unwired: 1 in, 1 out]
        n226 = call <vilib>:"NT Read String Array.vi"("Name"="/TestMode/TestList") -> ("String Array"=w381:string[])  [unwired: 9 in, 1 out]
        n227 = Build Array (concatenate)("Select the test to run...", w381) -> (w380:string[])
        n228 = property on="Test Name" class="Ring (strict)"("Strings []"=w380) -> ()  [unwired: 2 in, 2 out]
      }
      event "Test Name": Value Change {
        w384 = FALSE ("Visible")
        # "Tell the robot the test name to run"
        n229 = event-data() -> ("NewVal"=w388:u16)  [unwired: 1 in]
        n230 = property on="Test Name" class="Ring (strict)"() -> ("Strings []"=w389:string[])  [unwired: 2 in, 2 out]
        n231 = local write "Progress"(T7 {"Test Progress"=0, "Test Progress Text"=""} ("Progress")) -> ()
        n232 = Index Array(array=w389, index=w388) -> (element=w387:string)
        n233 = call <vilib>:"NT Write String.vi"("String"=w387, "Name"="/TestMode/TestName") -> ()  [unwired: 9 in, 1 out]
        n234 = property on="Progress" class="Clust (strict)"("Visible"=TRUE) -> ()  [unwired: 2 in, 2 out]
        n235 = property on="Motor" class="Clust (strict)"("Visible"=w384) -> ()  [unwired: 2 in, 2 out]
        n236 = property on="Test Slider" class="Slide (strict)"("Visible"=w384) -> ()  [unwired: 2 in, 2 out]
        n237 = property on="On/Off" class="Bool (strict)"("Visible"=w384) -> ()  [unwired: 2 in, 2 out]
        n238 = property on="Rev/Fwd" class="Clust (strict)"("Visible"=w384) -> ()  [unwired: 2 in, 2 out]
        n239 = property on="Test Ring" class="Ring (strict)"("Visible"=w384) -> ()  [unwired: 2 in, 2 out]
      }
      event "Select Auto": Mouse Enter {
        # "Populate the combo box with the list of autonomous options"
        n240 = event-data() -> ()  [unwired: 1 in, 1 out]
        n241 = call <vilib>:"NT Read String Array.vi"("Name"="Auto List") -> ("String Array"=w391:string[])  [unwired: 9 in, 1 out]
        n242 = property on="Select Auto" class="CmbBox"("Strings[]"=w391) -> ()  [unwired: 2 in, 2 out]
      }
      event "Select Auto": Value Change {
        # "User modified the Auto Selection. Write to NT variable so robot knows."
        n243 = event-data() -> ("NewVal"=w395:string)  [unwired: 1 in]
        n244 = call <vilib>:"NT Write String.vi"("String"=w395, "Name"="Auto Selector") -> ()  [unwired: 9 in, 1 out]
      }
      event "Command Selection": Value Change {
        # "Get the params and show in table"
        n245 = event-data() -> ("NewVal"=w402:i32)  [unwired: 1 in]
        n246 = property on="Command Selection" class="MCListbox (strict)"() -> ("ItemNames"=w400:string[][])  [unwired: 2 in, 2 out]
        n247 = call <vilib>:"WPI_DashboardUpdate Command Params.vi"("NewVal"=w402, "Commands"=w400, "Param Tbl"=w401) -> ()  [unwired: 8 in, 1 out]
      }
      event "Execute Command": Value Change {
        # "Started one, Unique ID holds\nresponse"
        n248 = event-data() -> ()  [unwired: 1 in, 1 out]
        n249 = property on="Command Selection" class="MCListbox (strict)"() -> ("ItemNames"=w414:string[][])  [unwired: 2 in, 2 out]
        n250 = Index Array(array=w414, index (row)="Command Selection", index (col)=0) -> (element=w412:string)
        n251 = call <vilib>:"Invoke Commands.vi"("Command Params"="Command Params", "Function Name"=w412) -> ("Params"=w408:u8, "Started"=w407:bool)  [unwired: 7 in, 1 out]
        n252 = Array Subset(array="Command Params", length (row)=w408) -> (w409:string[][])  [unwired: 3 in]
        n253 = Select(t="Executing" ("Cmd Status"), s=w407, f="" ("Cmd Status")) -> (s? t:f=→"Cmd Status":string)
      }
      event "Command Selection": Double Click {
        n254 = event-data() -> ("Row"=w424:i32)  [unwired: 1 in]
        n255 = property on="Command Selection" class="MCListbox (strict)"() -> ("ItemNames"=w427:string[][])  [unwired: 2 in, 2 out]
        n256 = local read "Command Params"() -> (w422:string[][])
        n257 = Index Array(array=w427, index (row)=w424, index (col)=0) -> (element=w425:string)
        n258 = call <vilib>:"Invoke Commands.vi"("Command Params"=w422, "Function Name"=w425) -> ("Params"=w421:u8, "Started"=w416:bool)  [unwired: 7 in, 1 out]
        n259 = Array Subset(array=w422, length (row)=w421) -> (w420:string[][])  [unwired: 3 in]
        n260 = Select(t="Executing" ("Cmd Status"), s=w416, f="" ("Cmd Status")) -> (s? t:f=w417:string)
        n261 = local write "Cmd Status"(w417) -> ()
      }
      event "CheckList": Double Click {
        # "Shift clears all"
        # "Update symbols on the listbox"
        n262 = event-data() -> ("PlatMods.Shift"=w430:bool, "Row"=w432:i32)  [unwired: 1 in]
        n263 = case shown="True" w430 {
          tunnel: w432 -> [w436 _]
          tunnel: 1 -> [w435 _]
          frame False {
            n264 = property on="CheckList" class="LstBox (strict)"() -> ("Item Symbols"=w434:i32[])  [unwired: 2 in, 2 out]
            n265 = Replace Array Subset(array=w434, new element=w435, index=w436) -> (w433:i32[])
            n266 = property on="CheckList" class="LstBox (strict)"("Item Symbols"=w433) -> ()  [unwired: 2 in, 2 out]
          }
          frame True {
            w437 = 0 ("Top Row")
            n267 = property on="CheckList" class="LstBox (strict)"() -> ("Number of Rows"=w439:u32)  [unwired: 2 in, 2 out]
            n268 = Initialize Array(0, w439) -> (w438:i32[])
            n269 = property on="CheckList" class="LstBox (strict)"("Top Row"=w437, "Value"=w437, "Item Symbols"=w438) -> ()  [unwired: 2 in, 2 out]
          }
        }
      }
      event "CheckList": Key Down {
        # "Update symbols on the listbox\nLeft and right keys check and uncheck"
        n270 = event-data() -> ("VKey"=w444:T22)  [unwired: 1 in]
        n271 = case shown="\"Left\", \"Right\"" w444 {
          selector: w444 -> [w449 _]
          tunnel: eventvkey."Left" ("VKey") -> [w447 _]
          frame "Left", "Right" {
            n272 = Equal?(x=w447, y=w449) -> (x = y?=w448:bool)
            n273 = Select(t=0, s=w448, f=1) -> (s? t:f=w450:i32)
            n274 = property on="CheckList" class="LstBox (strict)"() -> ("Item Symbols"=w453:i32[])  [unwired: 2 in, 2 out]
            n275 = Replace Array Subset(array=w453, new element=w450, index="CheckList") -> (w452:i32[])
            n276 = property on="CheckList" class="LstBox (strict)"("Item Symbols"=w452) -> ()  [unwired: 2 in, 2 out]
          }
          frame Default {
          }
        }
      }
      event "DB Camera Config": Value Change {
        # "Show or hide the cluster of controls, store in ini file"
        n277 = event-data() -> ("NewVal"=w458:bool)  [unwired: 1 in]
        n278 = case shown="False" w458 {
          tunnel: w457 -> [w467 _]
          tunnel: [w460 w478] -> w456
          tunnel: w455 -> [w459 w478]
          frame False {
            w474 = "Camera"
            w477 = FALSE ("Visible")
            n279 = local read "Camera Settings"() -> (w466:T2)
            n280 = Index Array(array=w467) -> (element=w470:cluster{string[]})  [unwired: 1 in]
            n281 = Unbundle(w466) -> ("Frame Rate"=w465:i32, "Compression"=w464:i32, "Size"=w468:u16)
            n282 = Unbundle(w470) -> (w469:string[])
            n283 = Index Array(array=w469, index=w468) -> (element=w463:string)
            n284 = call-poly <vilib>:"Write Key.vi"("section"=w474, "value"=w463, "key"="Size", "refnum"=w459) -> ("refnum out"=w476:T20)  [unwired: 2 in, 5 out]
            n285 = call-poly <vilib>:"Write Key.vi"("section"=w474, "value"=w465, "key"="FrameRate", "refnum"=w476) -> ("refnum out"=w475:T20)  [unwired: 1 in, 6 out]
            n286 = property on="Camera Settings" class="Clust (strict)"("Visible"=w477) -> ()  [unwired: 2 in, 2 out]
            n287 = local write "DB Camera Config"(w477) -> ()
            n288 = call-poly <vilib>:"Write Key.vi"("section"=w474, "value"=w464, "key"="Compression", "refnum"=w475) -> ("refnum out"=w461:T20)  [unwired: 1 in, 6 out]
            n289 = call <vilib>:"Close Config Data.vi"("refnum"=w461) -> ("file path"=w462:path)  [unwired: 2 in, 8 out]
            n290 = call <vilib>:"Open Config Data.vi"("configuration file path"=w462) -> ("refnum"=w460:T20)  [unwired: 8 in, 2 out]
          }
          frame True {
            n291 = property on="Camera Settings" class="Clust (strict)"("Visible"=TRUE) -> ()  [unwired: 2 in, 2 out]
          }
        }
      }
      event "Camera Settings": Value Change {
        # "Update summary string when any elements of DB camera change"
        n292 = event-data() -> ("NewVal"=w492:T2)  [unwired: 1 in]
        n293 = Index Array(array=w488) -> (element=w487:cluster{string[]})  [unwired: 1 in]
        n294 = Unbundle(w492) -> ("Frame Rate"=w483:i32, "Compression"=w482:i32, "Size"=w485:u16)
        n295 = Unbundle(w487) -> (w486:string[])
        n296 = Index Array(array=w486, index=w485) -> (element=w484:string)
        n297 = Format Into String(format string="%s   %dfps   %d%%", w484, w483, w482) -> (resulting string=w489:string)  [unwired: 2 in, 1 out]
        n298 = Build Array(w489) -> (w490:string[])
        n299 = property on="DB Camera Config" class="Bool (strict)"("Strings [4]"=w490) -> ()  [unwired: 2 in, 2 out]
      }
      event "Motor.Enable": Value Change {
        # "When the test mode otor enable helper is set, update that\ntree row item's value"
        n300 = event-data() -> ("NewVal"=w499:bool)  [unwired: 1 in]
        n301 = Unbundle("Motor") -> ("Value"=w498:dbl)  [unwired: 1 out]
        n302 = Select(t=w498, s=w499, f=0.0) -> (s? t:f=w496:dbl)
        n303 = call <vilib>:"NT Write Number.vi"("Numeric"=w496, "Name"=w495) -> ()  [unwired: 9 in, 1 out]
      }
      event "Test Slider": Value Change {
        # "When the test mode slider helper is set, update that\ntree row item's value"
        n304 = event-data() -> ("NewVal"=w503:dbl)  [unwired: 1 in]
        n305 = call <vilib>:"NT Write Number.vi"("Numeric"=w503, "Name"=w504) -> ()  [unwired: 9 in, 1 out]
      }
      event "On/Off": Value Change {
        # "When the test mode on/off helper value is set, update that\ntree row item's value"
        n306 = event-data() -> ("NewVal"=w509:bool)  [unwired: 1 in]
        n307 = Boolean To (0,1)(Boolean=w509) -> (0, 1=w508:i16)
        n308 = call <vilib>:"NT Write Number.vi"("Numeric"=w508, "Name"=w507) -> ()  [unwired: 9 in, 1 out]
      }
      event "Rev/Fwd": Value Change {
        # "When the test mode helper value for relays is set, update that\ntree row item's value"
        n309 = event-data() -> ("NewVal.Forward"=w518:bool, "NewVal.Reverse"=w517:bool)  [unwired: 1 in]
        n310 = Boolean To (0,1)(Boolean=w518) -> (0, 1=w514:i16)
        n311 = Boolean To (0,1)(Boolean=w517) -> (0, 1=w516:i16)
        n312 = Negate(x=w516) -> (-x=w515:i16)
        n313 = Add(x=w514, y=w515) -> (x+y=w513:i16)
        n314 = call <vilib>:"NT Write Number.vi"("Numeric"=w513, "Name"=w512) -> ()  [unwired: 9 in, 1 out]
      }
      event "Test Ring": Value Change {
        # "When a test mode helper value is selected from the ring,\nset the tree item's variable to the string value"
        n315 = event-data() -> ("NewVal"=w523:u16)  [unwired: 1 in]
        n316 = property on="Test Ring" class="Ring (strict)"() -> ("Strings []"=w524:string[])  [unwired: 2 in, 2 out]
        n317 = Index Array(array=w524, index=w523) -> (element=w522:string)
        n318 = call <vilib>:"NT Write String.vi"("String"=w522, "Name"=w521) -> ()  [unwired: 9 in, 1 out]
      }
      event "Rec Mode": Value Change {
        # "Update globals for recording mode and path to read log from.\nClear when logging and let NetworkTables set path for vision to\nuse."
        n319 = event-data() -> ("NewVal"=w536:enum32{"Stop", "Record", "Playback"})  [unwired: 1 in]
        n320 = global write "WPI_DashboardLogging Global.vi" "Logging Filename"(path "") -> ()
        n321 = global write "WPI_DashboardLogging Global.vi" "Recording"(w536) -> ()
        n322 = case shown="\"Playback\"" w536 {
          tunnel: w535 -> [_ w538 w547]
          tunnel: [_ _ w546] -> w532
          tunnel: [_ _ w545] -> _
          tunnel: w530 -> [_ _ w543]
          tunnel: cluster{i32, i32} {-250, 170} -> [_ _ w542]
          tunnel: [_ _ T23 {"Image Size"=TRUE, "Image Type"=TRUE, "Pixel Value"=TRUE, "ROI Information"=TRUE, "Zoom Factor"=FALSE} ("Image Information Shown:All Elements")] -> w528
          tunnel: [_ _ TRUE ("Zoom Factor")] -> w527
          tunnel: w526 -> [_ _ w539]
          frame Default {
          }
          frame "Stop", "Record" {
            # "Place Window too"
            n323 = invoke class="VI" method="FP.Close"(reference=w538) -> (reference out=w537:refnum<vi>)  [unwired: 2 in, 2 out]
            n324 = invoke class="VI" method="Abort VI"(reference=w537) -> ()  [unwired: 2 in, 3 out]
          }
          frame "Playback" {
            n325 = call "Open Playback Panel.vi"("Offset"=w542, "DB VI Ref"=w543, "Playback in"=w547) -> ("Playback out"=w544:refnum<vi>)  [unwired: 8 in]
            n326 = register-events(w544, w539) -> (reference out=w546:refnum<event-registration>, error out=w545:errorcluster)  [unwired: 2 in]
          }
        }
        n327 = property on="Camera Image" class="ImageControl"("Image Information Shown"=w528, "Image Information Visible"=w527) -> ()  [unwired: 2 in, 2 out]
        n328 = call <vilib>:"WPI_DashboardNT Log FieldName Cache.vi"("Operation"=enum16{"Lookup/Add", "Index", "Clear"}."Clear") -> ()  [unwired: 8 in, 3 out]
      }
      event Panel Close {
        w549 = enum32{"Stop", "Record", "Playback"}."Stop" ("Rec Mode")
        # "Playback window has been closed, abort"
        n329 = event-data() -> ()  [unwired: 1 in, 4 out]
        n330 = local write "Rec Mode"(w549) -> ()
        n331 = global write "WPI_DashboardLogging Global.vi" "Recording"(w549) -> ()
      }
      event Panel Close {
        # "Abort playback window and ourself"
        n332 = event-data() -> ()  [unwired: 1 in, 4 out]
        n333 = invoke class="VI" method="FP.Close"(reference=w555) -> (reference out=w554:refnum<vi>)  [unwired: 2 in, 2 out]
        n334 = invoke class="VI" method="Abort VI"(reference=w554) -> (error out=w553:errorcluster)  [unwired: 2 in, 2 out]
        n335 = invoke class="VI" method="Abort VI"(error in=w553) -> ()  [unwired: 2 in, 3 out]
      }
      event User Event {
        n336 = event-data() -> ("IDs"=w563:cluster{"RPC field ID":u16, "Unique ID":u16}, "String"=w562:string)  [unwired: 1 in]
        n337 = Bundle("IDs"=w563, "String"=w562) -> (w561:T9)  [unwired: 1 in]
        n338 = call <vilib>:"Retrieve RPC Response.vi"("RPC Response"=w561) -> ("Output"=w558:string[][])  [unwired: 10 in]
        n339 = Build Array (concatenate)(w556, w558) -> (w557:string[][])
        n340 = local write "Command Params"(w557) -> ()
        n341 = local write "Cmd Status"("" ("Cmd Status")) -> ()
      }
      event "Vision": Value Change {
        # "Enable/Disable Compression slider.\nHW USB is hard-coded into the camera"
        n342 = event-data() -> ("NewVal"=w570:u16)  [unwired: 1 in]
        n343 = Equal?(x=w570, y=u32 2 ("milliseconds to wait")) -> (x = y?=w568:bool)
        n344 = Select(t=T24."Disabled and Grayed Out" ("Disabled"), s=w568, f=T24."Enabled" ("Disabled")) -> (s? t:f=w565:T24)
        n345 = property on="Compression" class="Slide (strict)"("DisabledEnum"=w565) -> ()  [unwired: 2 in, 2 out]
      }
      event "Tree": Double Click {
        n346 = event-data() -> ("PlatMods"=w575:T27, "Tag"=w574:string)  [unwired: 1 in]
        n347 = Unbundle(w575) -> ("Shift"=w573:bool)  [unwired: 4 out]
        n348 = Not(x=w573) -> (.not. x?=w572:bool)
        n349 = call <vilib>:"NT Update Persistence.vi"("Persistence"=w572, "Name"=w574) -> ()  [unwired: 9 in, 1 out]
      }
    }
  }
  n350 = while {
    tunnel: w54 -> [w579]
    i -> [w582]
    stop <- FALSE stop-if-true
    n351 = Wait (ms)(milliseconds to wait=u32 100) -> ()  [unwired: 1 out]
    n352 = case shown="\"Stop\", Default" "Rec Mode" {
      tunnel: w582 -> [_ _ w597]
      tunnel: [u32 2829099 ("Base Color") u32 11141120 ("Target Color") w586] -> w578
      frame "Stop", Default {
        # "Reset the color, extra updates don't cost much"
      }
      frame "Record" {
      }
      frame "Playback" {
        # "Playback"
        n353 = Quotient & Remainder(x=w597, y=u32 50 ("milliseconds to wait")) -> (x-y*floor(x/y)=w593:u32)  [unwired: 1 out]
        n354 = Divide(x=w593, y=u32 50 ("milliseconds to wait")) -> (x/y=w590:dbl)
        n355 = Multiply(x=6.283185307179586, y=w590) -> (x*y=w595:dbl)
        n356 = Sine(x=w595) -> (sin(x)=w594:dbl)
        n357 = Absolute Value(x=w594) -> (abs(x)=w587:dbl)
        n358 = call "Interpolate RGB Color.vi"("Proportion"=w587, "Target Color"=u32 30976, "Base Color"=u32 2829099) -> ("Result Color"=w586:u32)  [unwired: 8 in]
      }
    }
    n359 = property class="Pane"(reference=w579, "PaneColor"=w578) -> ()  [unwired: 1 in, 2 out]
  }
  n360 = Less?(x=w4, y=60.0) -> (x < y?=→"gauche fort 2":bool)
  n361 = Greater?(x=w4, y=110.0) -> (0:→"gauche rapide 2":bool)
  n362 = local write "Dashboard Tab"(T1."Drive" ("Dashboard Tab")) -> ()
  n363 = property on="On/Off" class="Bool (strict)"("Visible"=w22) -> ()  [unwired: 2 in, 2 out]
  n364 = property on="Motor" class="Clust (strict)"("Visible"=w22) -> ()  [unwired: 2 in, 2 out]
  n365 = property on="Progress" class="Clust (strict)"("Visible"=w22) -> ()  [unwired: 2 in, 2 out]
  n366 = property on="Test Ring" class="Ring (strict)"("Visible"=w22) -> ()  [unwired: 2 in, 2 out]
  n367 = property on="Rev/Fwd" class="Clust (strict)"("Visible"=w22) -> ()  [unwired: 2 in, 2 out]
  n368 = property on="Camera Settings" class="Clust (strict)"("Visible"=w22) -> ()  [unwired: 2 in, 2 out]
  n369 = local write "DB Camera Config"(w22) -> ()
  n370 = local write "Command Params"(string[][] [] ("Command Params")) -> ()
  n371 = global write "WPI_DashboardLogging Global.vi" "Recording"(w48) -> ()
  n372 = local write "Rec Mode"(w48) -> ()
  n373 = while {
    tunnel: u16 1741 ("timeout ms (25000)") -> [w599]
    stop <- FALSE stop-if-true
    n374 = TCP Create Listener(10:w599) -> (0:w598:errorcluster, 3:w600:refnum<k5>)  [unwired: 4 in, 1 out]
    n375 = case shown="Error" w598 {
      selector: w598 -> [w602 _]
      tunnel: w600 -> [w603 _]
      frame No Error {
        n376 = while {
          tunnel: w603 -> [w606]
          tunnel: w602 -> [w605]
          stop <- FALSE stop-if-true
          n377 = TCP Wait On Listener(8:w605, 11:w606) -> (0:w607:errorcluster, 4:w608:refnum<k5>)  [unwired: 2 in, 3 out]
          n378 = local write "TCP"(w608) -> ()
          n379 = case shown="No Error" w607 {
            frame No Error {
            }
            frame Error {
              n380 = Wait (ms)(milliseconds to wait=u32 1000) -> ()  [unwired: 1 out]
            }
          }
        }
      }
      frame Error {
        n381 = Wait (ms)(milliseconds to wait=u32 1000) -> ()  [unwired: 1 out]
      }
    }
  }
  n382 = local write "Command Selection"(u16 0 ("milliseconds to wait")) -> ()
  n383 = call-poly <vilib>:"NT Read Value.vi"("Name"="Pelle bas") -> ()  [unwired: 9 in, 2 out]
